vi "Dequeue Table Buffer.vi"(8 "error in (no error)":errorcluster) -> (0 "error out":errorcluster, 3 "Data":string[][](array[string]))   [LabVIEW 2025, in "I2C Bus Monitor UI.lvlib"]
uses:
  I2C Bus Monitor UI.lvlib
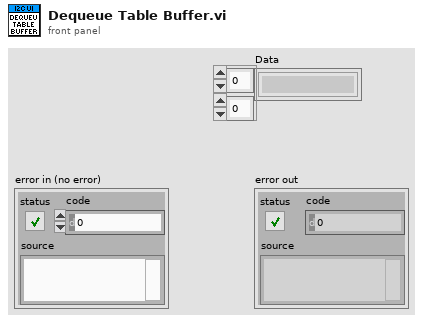
[diagram p1: front panel]
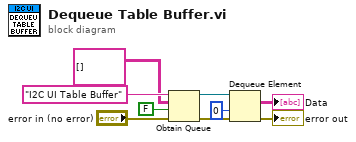
[diagram p0: block diagram]
diagram:
  n1 = Obtain Queue(name (unnamed)="I2C UI Table Buffer", element data type=string[][] [] ("I2C Messages"), create if not found? (T)=FALSE, error in (no error)="error in (no error)") -> (queue out=w3:refnum<queue>, error out=w6:errorcluster)  [unwired: 1 in, 1 out]
  n2 = Dequeue Element(queue=w3, timeout in ms (-1)=0, error in (no error)=w6) -> (element=→"Data":string[][], error out=→"error out":errorcluster)  [unwired: 2 out]
